vi "BouncerDAQinit.vi"(8 "error in (no error)":errorcluster) -> (0 "error out":errorcluster, 1 "Run Ratios":T2 {"LEC13/12" format="%_4e"; "DTfrac" format="%#_3g"; "DT" format="%#_3g"; "CountErr" format="%#_3g"; "d13C" format="%_4g"; "C13/12" format="%_4e"; "C14/12" format="%_4e"; "C14/13" format="%_3e"; "C12Cor" format="%_3e"; "C13" format="%_3e"; "C13H/L" format="%#_3g"}, 2 "Summary Data":T1, 3 "Block Data":T4, 5 "Run Parameters":T3={"Block time (s)"=1.0, "Max Runtime (s)"=10.0, "Max Counts"=10000, "C12 Limit"=-1.0, "Max BadBlocks"=100, "Tuning"=TRUE, "WarmupTime"=0.0, "Warmup"=FALSE} {"Block time (s)" min=0.0 max=100.0 step=0.1})   [LabVIEW 2013]
uses:
  ctl/BlockData.ctl
  ctl/RunParameters.ctl
  ctl/RunRatios.ctl
  ctl/SummaryData.ctl
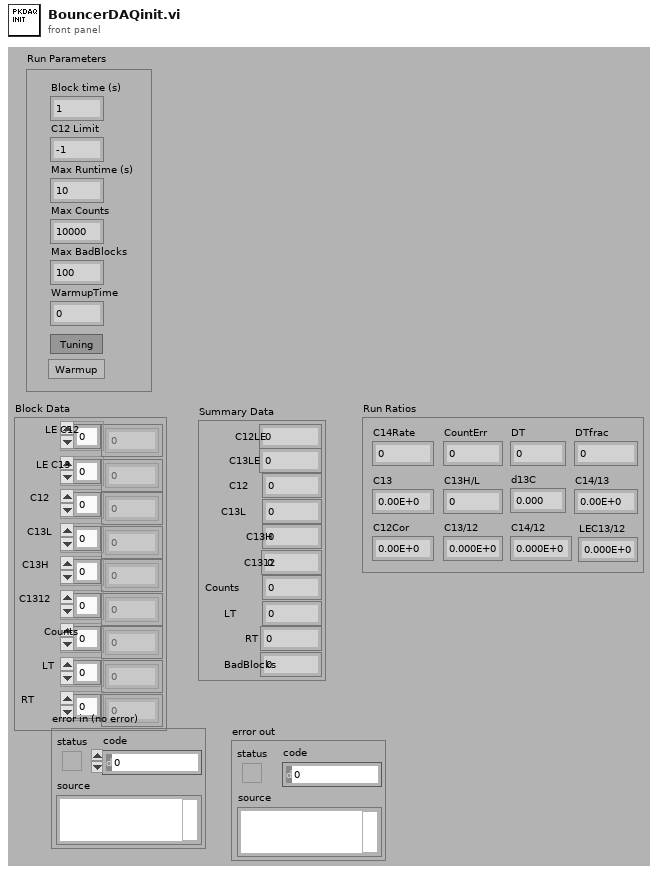
[diagram p1: front panel]
types:
  T1 = typedef "SummaryData.ctl" = cluster{"C12LE":dbl, "C13LE":dbl, "C12":dbl, "C13L":dbl, "C13H":dbl, "C1312":dbl, "Counts":u32, "LT":dbl, "RT":dbl, "BadBlocks":u8}
  T2 = typedef "RunRatios.ctl" = cluster{"C14Rate":dbl, "CountErr":dbl, "DT":dbl, "DTfrac":dbl, "C13":dbl, "C13H/L":dbl, "d13C":dbl, "C14/13":dbl, "C12Cor":dbl, "C13/12":dbl, "C14/12":dbl, "LEC13/12":dbl}
  T3 = typedef "RunParameters.ctl" = cluster{"Block time (s)":dbl, "Max Runtime (s)":dbl, "Max Counts":u32, "C12 Limit":dbl, "Max BadBlocks":u8, "Tuning":bool, "WarmupTime":dbl, "Warmup":bool}
  T4 = typedef "BlockData.ctl" = cluster{"LE C12":dbl[], "LE C13":dbl[], "C12":dbl[], "C13L":dbl[], "C13H":dbl[], "C1312":dbl[], "Counts":u32[], "LT":dbl[], "RT":dbl[]}
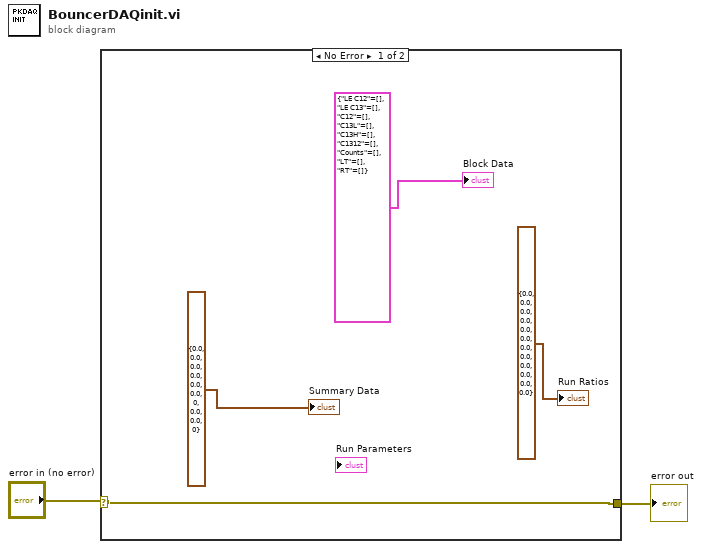
[diagram p0: block diagram]
diagram:
  n1 = case shown="No Error" "error in (no error)" {
    selector: "error in (no error)" -> [w6 w7]
    tunnel: [w6 w7] -> w2
    frame No Error {
      "Block Data" <- T4 {"LE C12"=[], "LE C13"=[], "C12"=[], "C13L"=[], "C13H"=[], "C1312"=[], "Counts"=[], "LT"=[], "RT"=[]} ("Block Data 2")
      "Run Ratios" <- T2 {"C14Rate"=0.0, "CountErr"=0.0, "DT"=0.0, "DTfrac"=0.0, "C13"=0.0, "C13H/L"=0.0, "d13C"=0.0, "C14/13"=0.0, "C12Cor"=0.0, "C13/12"=0.0, "C14/12"=0.0, "LEC13/12"=0.0} ("Run Ratios 2")
      "Summary Data" <- T1 {"C12LE"=0.0, "C13LE"=0.0, "C12"=0.0, "C13L"=0.0, "C13H"=0.0, "C1312"=0.0, "Counts"=0, "LT"=0.0, "RT"=0.0, "BadBlocks"=0} ("Summary Data 2")
    }
    frame Error {
    }
  }
  "error out" <- w2
